vi "Create Folder if Invalid Ref.vi"(7 "Name":string, 8 "Access Scope (none)":T1(ring), 9 "Parent":refnum<vi>, 10 "Library":refnum<vi>, 11 "Folder Ref In":refnum<vi>) -> (3 "Folder Ref":refnum<vi>)   [LabVIEW 2018, in "LVClassByRef.lvlib"]
uses:
  <resource>/Framework/Providers/LVClassByRef/LVClassByRef.lvlib
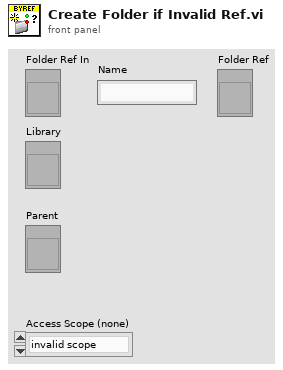
[diagram p1: front panel]
types:
  T1 = enum32{"invalid scope", "public", "private", "protected", "community"}
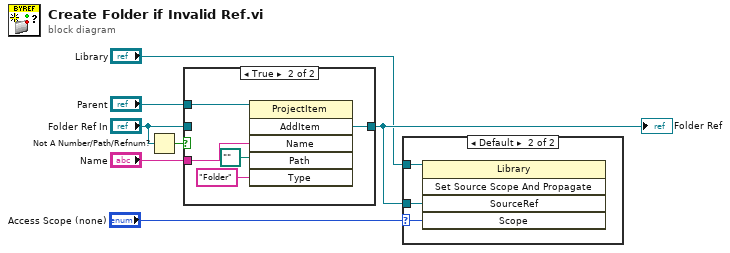
[diagram p0: block diagram]
diagram:
  n1 = Not A Number/Path/Refnum?(number/path/refnum="Folder Ref In") -> (NaN/Path/Refnum?=w7:bool)
  n2 = case shown="True" w7 {
    tunnel: "Name" -> [_ w12]
    tunnel: "Parent" -> [_ w13]
    tunnel: "Folder Ref In" -> [w8 _]
    tunnel: [w8 w10] -> w3
    frame False {
    }
    frame True {
      n3 = invoke class="ProjectItem" method="AddItem"(reference=w13, "Name"=w12, "Path"=path "", "Type"="Folder") -> ("AddItem"=w10:refnum<vi>)  [unwired: 2 in, 5 out]
    }
  }
  "Folder Ref" <- w3
  n4 = case shown="Default" "Access Scope (none)" {
    selector: "Access Scope (none)" -> [_ w15]
    tunnel: "Library" -> [_ w16]
    tunnel: w3 -> [_ w14]
    frame "invalid scope" {
    }
    frame Default {
      n5 = invoke class="Library" method="Set Source Scope And Propagate"(reference=w16, "SourceRef"=w14, "Scope"=w15) -> ()  [unwired: 2 in, 5 out]
    }
  }
